vi "octaViewer.vi"() -> ()   [LabVIEW 2017]
panel:
  out "Loaded":bool
  out "Loading":bool
  out "Current frame":string
  out "Image":T1(plugin-control)
  in  "Select frame":u16(c297)
  in  "stop":bool
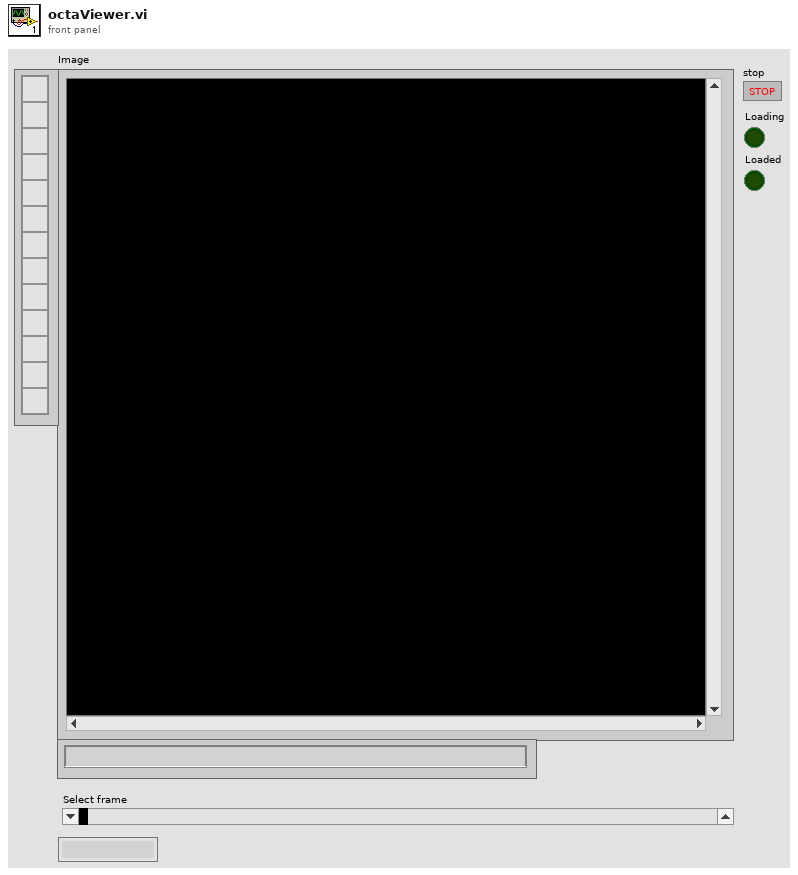
[diagram p1: front panel]
types:
  T1 = typedef "IMAQ Image.ctl" = refnum<image>
  T2 = enum16{"None", "On Hover", "On Key Focus", "On Hover or Key Focus"}
  T3 = typedef "Image Type" = u32
  T4 = enum16{"big-endian, network order", "native, host order", "little-endian"}
  T5 = enum16{"open", "replace", "create", "open or create", "replace or create", "replace or create with confirmation"}
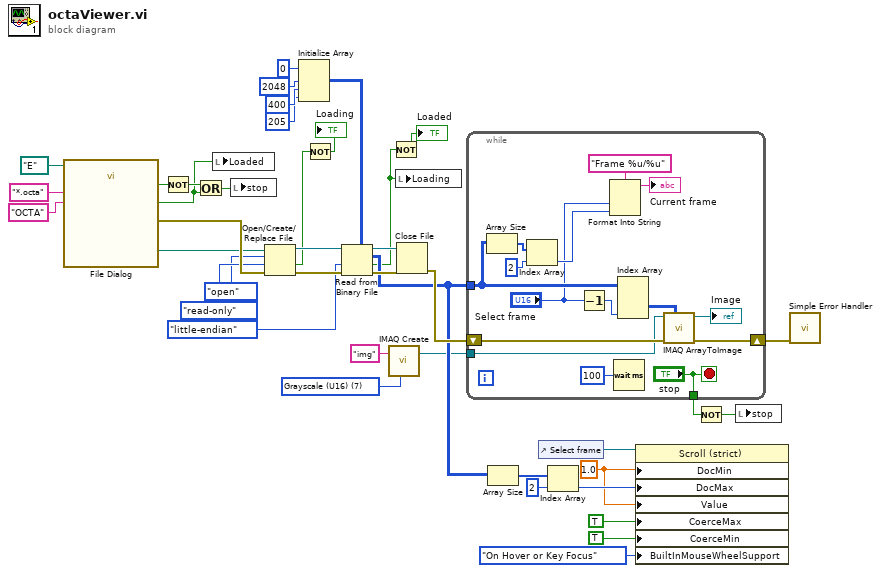
[diagram p0: block diagram]
diagram:
  w15 = 1.0 ("Doc Min")
  w24 = T3 7 items=["Grayscale (U8)", "Grayscale (I16)", "Grayscale (SGL)", "Complex (CSG)", "RGB (U32)", "HSL (U32)", "RGB (U64)", "Grayscale (U16)"] ("Image Type")
  n1 = call "File Dialog"("start path"=path "E:/", "pattern (all files)"="*.octa", "pattern label"="OCTA") -> ("selected path"=w33:path, "exists"=w35:bool, "cancelled"=w2:bool, "error out"=w34:errorcluster)  [unwired: 9 in]
  n2 = Not(x=w35) -> (.not. x?=w36:bool)
  n3 = Or(x=w36, y=w2) -> (x .or. y?=w3:bool)
  n4 = local write "Loaded"(w2) -> ()
  n5 = local write "stop"(w3) -> ()
  n6 = Open/Create/Replace File(file path (use dialog)=w33, error in=w34, operation (0:open)=T5."open", access (0:read/write)=enum16{"read/write", "read-only", "write-only"}."read-only") -> (refnum out=w37:refnum<file>, cancelled=w12:bool, error out=w38:errorcluster)  [unwired: 2 in]
  n7 = Initialize Array(u16 0 ("element"), 2048 ("dimension size"), 400 ("dimension size"), 205 ("dimension size")) -> (w4:u16[][][])
  n8 = Not(x=w12) -> (.not. x?=→"Loading":bool)
  n9 = Read from Binary File(5:w4, 8:w38, 9:T4."little-endian" ("byte order (0:big-endian, network order)"), 11:w37) -> (0:w40:errorcluster, 1:w9:bool, 2:w26:u16[][][], 3:w39:refnum<file>)  [unwired: 2 in]
  n10 = call "IMAQ Create"("Image Name"="img", "Image Type"=w24) -> ("New Image"=w23:T1)  [unwired: 3 in, 1 out]
  n11 = Not(x=w9) -> (.not. x?=→"Loaded":bool)
  n12 = local write "Loading"(w9) -> ()
  n13 = Close File(refnum=w39, error in=w40) -> (error out=w41:errorcluster)  [unwired: 1 out]
  n14 = while {
    tunnel: w26 -> [w48]
    shift-right: [w53] -> w22
    shift-left: w41 -> [w54]
    tunnel: w23 -> [w52]
    tunnel: ["stop"] -> w18
    stop <- "stop" stop-if-true
    n15 = Array Size(array=w48) -> (size(s)=w47:i32[])
    n16 = Index Array(array=w47, index=2) -> (element=w45:i32)
    n17 = Decrement(x="Select frame") -> (x-1=w43:u16)
    n18 = Format Into String(format string="Frame %u/%u", "Select frame", w45) -> (resulting string=→"Current frame":string)  [unwired: 2 in, 1 out]
    n19 = Wait (ms)(milliseconds to wait=u32 100) -> ()  [unwired: 1 out]
    n20 = Index Array(array=w48, index (dim 2)=w43) -> (element=w42:u16[][])  [unwired: 2 in]
    n21 = call "IMAQ ArrayToImage"("Image Pixels (U16)"=w42, "error in (no error)"=w54, "Image"=w52) -> ("error out"=w53:errorcluster, "Image Out"=→"Image":T1)  [unwired: 7 in]
  }
  n22 = Array Size(array=w26) -> (size(s)=w20:i32[])
  n23 = control-ref of="Select frame"() -> (w21:refnum<vi>)
  n24 = Index Array(array=w20, index=2) -> (element=w16:i32)
  n25 = property class="Scroll (strict)"(reference=w21, "DocMin"=w15, "DocMax"=w16, "Value"=w15, "CoerceMax"=TRUE ("Coerce Maximum Value"), "CoerceMin"=TRUE ("Coerce Minimum Value"), "BuiltInMouseWheelSupport"=T2."On Hover or Key Focus" ("Built-In Mouse Wheel Support")) -> ()  [unwired: 1 in, 2 out]
  n26 = Not(x=w18) -> (.not. x?=w17:bool)
  n27 = local write "stop"(w17) -> ()
  n28 = call <vilib>:"Simple Error Handler.vi"("error in (no error)"=w22) -> ()  [unwired: 4 in, 5 out]
